vi "InitHardware.vi"(8 "error in (no error)":errorcluster, 11 "ThorLabsCsCamera in":refnum<class "ThorLabsCsCamera.lvclass">) -> (0 "error out":errorcluster, 1 "bit depth":string, 2 "Image Type":T3 items=["Grayscale (U8)", "Grayscale (I16)", "Grayscale (SGL)", "Complex (CSG)", "RGB (U32)", "HSL (U32)", "RGB (U64)", "Grayscale (U16)"], 3 "ThorLabsCsCamera out":refnum<class "ThorLabsCsCamera.lvclass">)   [LabVIEW 2020, in "ThorLabsCsCamera.lvclass"]
uses:
  ThorLabsCsCamera.lvclass
  C:/GEECS/Developers Version/source/Device Drivers/Point Grey Camera/Point Grey Camera.lvclass
  Thorlabs VIs/Controls/Region of Interest.ctl
  Thorlabs VIs/Controls/Binning.ctl
  Point Grey Camera/Point Grey Camera.lvclass/Point Grey Camera.ctl
  ThorLabsCsCamera.lvclass/ThorLabsCsCamera.ctl
  Point Grey Camera/Read Settings 2.vi
  Point Grey Camera/Write Settings 2.vi
  Thorlabs VIs/SubVIs/Parameters Get & Set/Get Parameters/Get ROIAndBin.vi
  Thorlabs VIs/SubVIs/Parameters Get & Set/Get Parameters/Get SensorHeight_pixels.vi
  Thorlabs VIs/SubVIs/Parameters Get & Set/Get Parameters/Get SensorWidth_pixels.vi
  Thorlabs VIs/SubVIs/Parameters Get & Set/Set Parameters/Set ROIAndBin.vi
  Thorlabs VIs/SubVIs/Parameters Get & Set/Get Parameters/Get CameraSensorType.vi
panel:
  out "Binning 2":T1
  out "Region of Interest 2":T2={"Origin - X"=0, "Origin - Y"=0, "Width"=1392, "Height"=1040}
  out "SensorHeight_pixels":u32
  out "SensorWidth_pixels":u32
  out "Binning":T1
  out "Region of Interest":T2={"Origin - X"=0, "Origin - Y"=0, "Width"=1392, "Height"=1040}
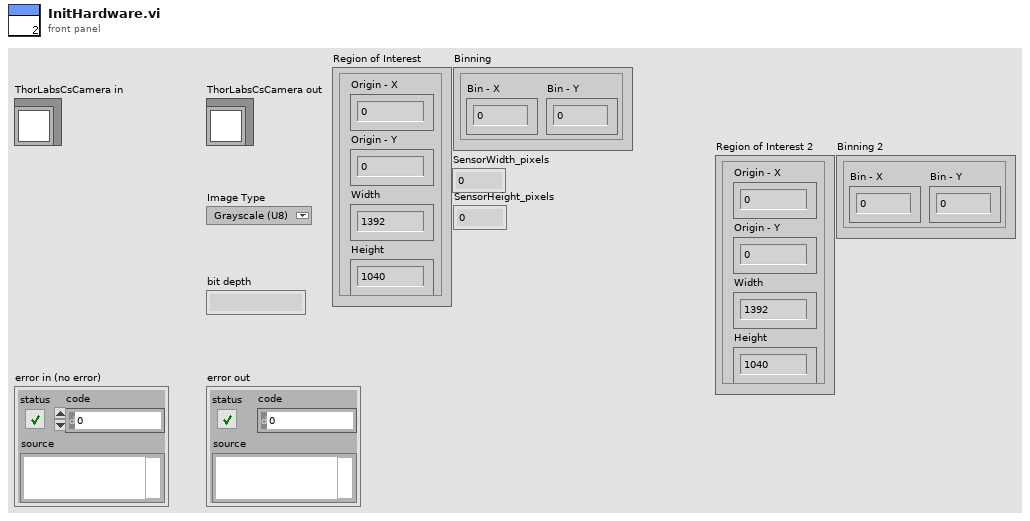
[diagram p1: front panel]
types:
  T1 = typedef "Binning.ctl" = cluster{"Bin - X":u32, "Bin - Y":u32}
  T2 = typedef "Region of Interest.ctl" = cluster{"Origin - X":u32, "Origin - Y":u32, "Width":u32, "Height":u32}
  T3 = typedef "Image Type" = u32
  T4 = typedef "Point Grey Camera.lvclass/SettingsTypdef.ctl" = cluster{"Trigger":T5, "Gain":cluster{"Value":dbl, "Min":dbl, "Max":dbl, "StepSize":dbl, "Tolerance":dbl, "valueactual":dbl}, "Exposure":cluster{"Value":dbl, "Min":dbl, "Max":dbl, "StepSize":dbl, "Tolerance":dbl, "valueactual":dbl}, "Timeout":cluster{"Value":dbl, "Min":dbl, "Max":dbl, "StepSize":dbl, "Tolerance":dbl, "valueactual":dbl}, "LocalSavingPath":path, "Save":T5, "TriggerDelay":cluster{"Value":dbl, "Min":dbl, "Max":dbl, "StepSize":dbl, "Tolerance":dbl, "valueactual":dbl}, "CamSession":string, "ROI":T6, "MaxGUIPixel":cluster{"Value":dbl, "Min":dbl, "Max":dbl, "StepSize":dbl, "Tolerance":dbl, "valueactual":dbl}, "Target":cluster{"X":cluster{"Value":dbl, "Min":dbl, "Max":dbl, "StepSize":dbl, "Tolerance":dbl, "valueactual":dbl}, "Y":cluster{"Value":dbl, "Min":dbl, "Max":dbl, "StepSize":dbl, "Tolerance":dbl, "valueactual":dbl}}, "Analysis":T5, "maxshot#":dbl, "SpatialCalibration":cluster{"Value":dbl, "Min":dbl, "Max":dbl, "StepSize":dbl, "Tolerance":dbl, "valueactual":dbl}, "roistatus":T5, "Lineout":T5, "AnalysisThreshold":cluster{"Value":dbl, "Min":dbl, "Max":dbl, "StepSize":dbl, "Tolerance":dbl, "valueactual":dbl}, "TargetSize":cluster{"X":cluster{"Value":dbl, "Min":dbl, "Max":dbl, "StepSize":dbl, "Tolerance":dbl, "valueactual":dbl}, "Y":cluster{"Value":dbl, "Min":dbl, "Max":dbl, "StepSize":dbl, "Tolerance":dbl, "valueactual":dbl}}, "Simulation":T5, "SpatialCalibrationY":cluster{"Value":dbl, "Min":dbl, "Max":dbl, "StepSize":dbl, "Tolerance":dbl, "valueactual":dbl}, "Target2":cluster{"X":cluster{"Value":dbl, "Min":dbl, "Max":dbl, "StepSize":dbl, "Tolerance":dbl, "valueactual":dbl}, "Y":cluster{"Value":dbl, "Min":dbl, "Max":dbl, "StepSize":dbl, "Tolerance":dbl, "valueactual":dbl}}, "Target2Size":cluster{"X":cluster{"Value":dbl, "Min":dbl, "Max":dbl, "StepSize":dbl, "Tolerance":dbl, "valueactual":dbl}, "Y":cluster{"Value":dbl, "Min":dbl, "Max":dbl, "StepSize":dbl, "Tolerance":dbl, "valueactual":dbl}}, "Crosshair":cluster{"Label1":string, "Label2":string}, "Max2ndMomRadius":cluster{"Value":dbl, "Min":dbl, "Max":dbl, "StepSize":dbl, "Tolerance":dbl, "valueactual":dbl}, "SaveType":T7, "BackgroundPath":path, "GUI8bit":T5, "GUICompression":T5, "CompressionQuality":cluster{"Value":dbl, "Min":dbl, "Max":dbl, "StepSize":dbl, "Tolerance":dbl, "valueactual":dbl}, "SaveAsync":T5, "PerspectivePath":path, "PerspectiveCorrectGUI":T5, "BlackLevel":cluster{"Value":dbl, "Min":dbl, "Max":dbl, "StepSize":dbl, "Tolerance":dbl, "valueactual":dbl}, "TargetBP":cluster{"X":cluster{"Value":dbl, "Min":dbl, "Max":dbl, "StepSize":dbl, "Tolerance":dbl, "valueactual":dbl}, "Y":cluster{"Value":dbl, "Min":dbl, "Max":dbl, "StepSize":dbl, "Tolerance":dbl, "valueactual":dbl}}, "PythonAnalysis":T5, "PythonFunctionName":string, "PythonLineout":T5, "PythonVersion":string, "GEECSBuildsPath":path, "DisplayPythonProcessedImage":T5, "PythonModuleName":string, "AnalysisThresholdHigh":cluster{"Value":dbl, "Min":dbl, "Max":dbl, "StepSize":dbl, "Tolerance":dbl, "valueactual":dbl}, "AnalysisMedianRank":cluster{"Value":dbl, "Min":dbl, "Max":dbl, "StepSize":dbl, "Tolerance":dbl, "valueactual":dbl}, "ClockSpeed":cluster{"Value":dbl, "Min":dbl, "Max":dbl, "StepSize":dbl, "Tolerance":dbl, "valueactual":dbl}, "AutoTrigger":T5, "AutoTriggerLevelMeanCounts":cluster{"Value":dbl, "Min":dbl, "Max":dbl, "StepSize":dbl, "Tolerance":dbl, "valueactual":dbl}, "AnalysisROILeft":cluster{"Value":dbl, "Min":dbl, "Max":dbl, "StepSize":dbl, "Tolerance":dbl, "valueactual":dbl}, "AnalysisROIRight":cluster{"Value":dbl, "Min":dbl, "Max":dbl, "StepSize":dbl, "Tolerance":dbl, "valueactual":dbl}, "AnalysisROITop":cluster{"Value":dbl, "Min":dbl, "Max":dbl, "StepSize":dbl, "Tolerance":dbl, "valueactual":dbl}, "AnalysisROIBottom":cluster{"Value":dbl, "Min":dbl, "Max":dbl, "StepSize":dbl, "Tolerance":dbl, "valueactual":dbl}, "AnalysisROI":T5, "UseSoftwareTrigger":T5, "UDPtrigger":T5, "AutoTriggerLevelMaxCounts":cluster{"Value":dbl, "Min":dbl, "Max":dbl, "StepSize":dbl, "Tolerance":dbl, "valueactual":dbl}}
  T5 = typedef "OnOffTypeDef.ctl" = enum16{"off", "on"}
  T6 = typedef "ROI_TypDef.ctl" = cluster{"Width":cluster{"Value":dbl, "Min":dbl, "Max":dbl, "StepSize":dbl, "Tolerance":dbl, "valueactual":dbl}, "Height":cluster{"Value":dbl, "Min":dbl, "Max":dbl, "StepSize":dbl, "Tolerance":dbl, "valueactual":dbl}, "OffsetX":cluster{"Value":dbl, "Min":dbl, "Max":dbl, "StepSize":dbl, "Tolerance":dbl, "valueactual":dbl}, "OffsetY":cluster{"Value":dbl, "Min":dbl, "Max":dbl, "StepSize":dbl, "Tolerance":dbl, "valueactual":dbl}}
  T7 = typedef "Image save type.ctl" = enum16{"PNG", "BMP", "JPEG", "TDMS", "hdf5"}
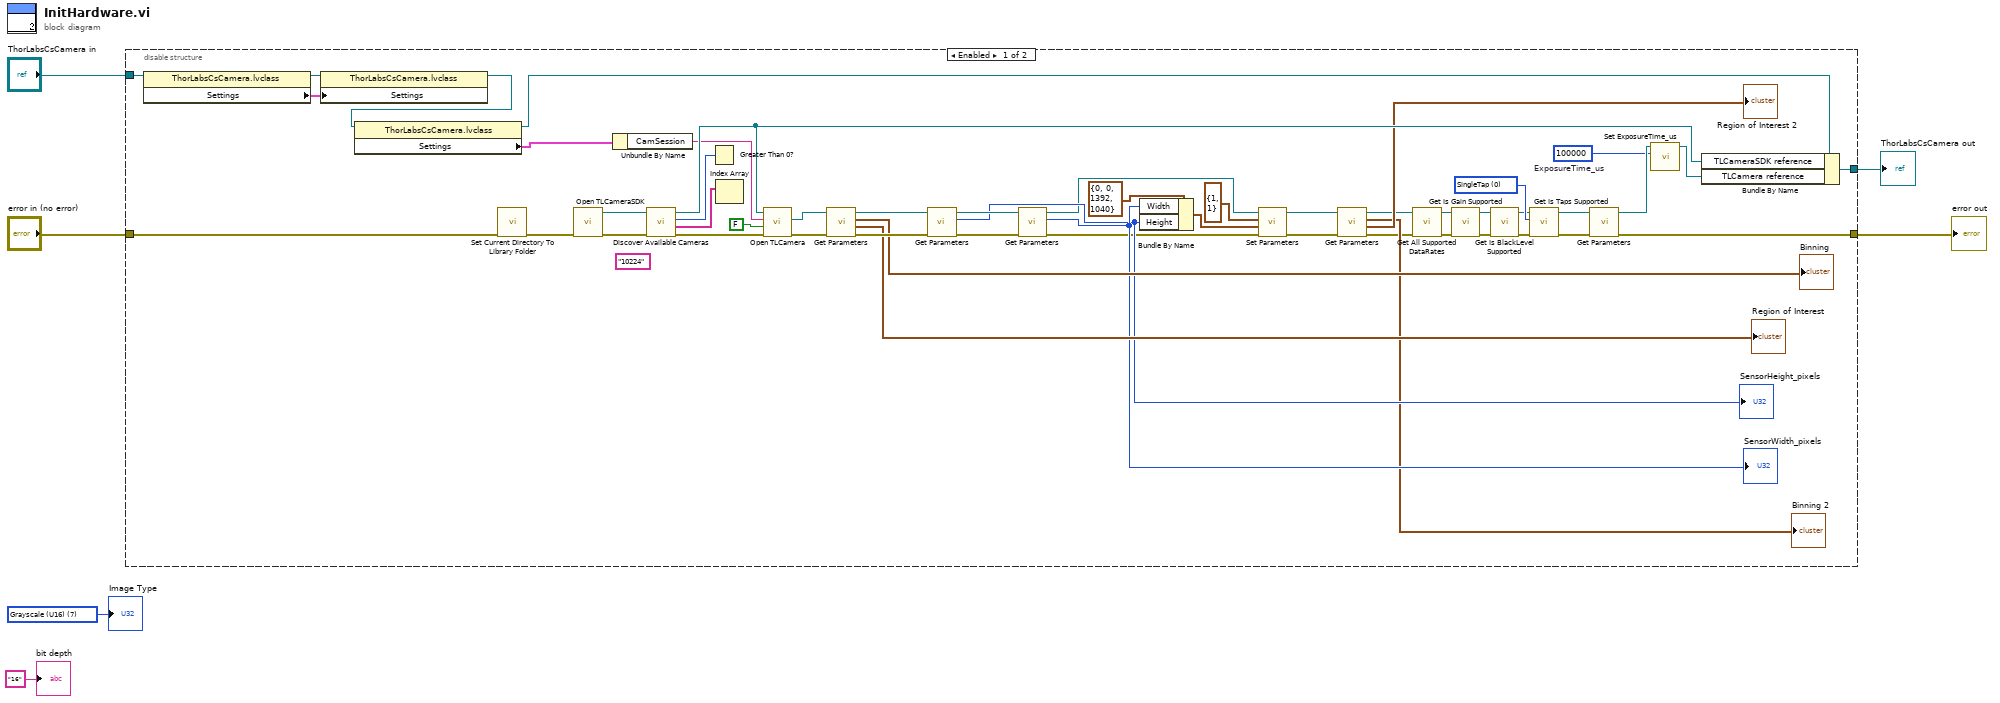
[diagram p0: block diagram]
diagram:
  w1 = T3 7 items=["Grayscale (U8)", "Grayscale (I16)", "Grayscale (SGL)", "Complex (CSG)", "RGB (U32)", "HSL (U32)", "RGB (U64)", "Grayscale (U16)"] ("Image Type")
  n1 = disable-structure shown="Enabled" {
    disable-tunnel: "error in (no error)" -> [w51 w58]
    disable-tunnel: "ThorLabsCsCamera in" -> [w35 w59]
    disable-tunnel: [w30 w59] -> w4
    disable-tunnel: [w29 w58] -> w3
    frame Enabled {
      (unwired) "10224" ("CamSession")
      w26 = u32 100000  # ExposureTime_us
      w44 = 0 items=["SingleTap", "DualTap", "QuadTap"] ("Taps")
      n2 = property class="ThorLabsCsCamera.lvclass"(reference=w35) -> (reference out=w56:refnum<class "ThorLabsCsCamera.lvclass">, "Settings"=w57:T4)  [unwired: 1 in, 1 out]
      n3 = property class="ThorLabsCsCamera.lvclass"(reference=w56, "Settings"=w57) -> (reference out=w9:refnum<class "ThorLabsCsCamera.lvclass">)  [unwired: 1 in, 1 out]
      n4 = property class="ThorLabsCsCamera.lvclass"(reference=w9) -> (reference out=w8:refnum<class "ThorLabsCsCamera.lvclass">, "Settings"=w10:T4)  [unwired: 1 in, 1 out]
      n5 = call "Set Current Directory To Library Folder.vi"("error in (no error)"=w51) -> ("error out"=w52:errorcluster)  [unwired: 10 in]
      n6 = call "Open TLCameraSDK.vi"("error in (no error)"=w52) -> ("error out"=w54:errorcluster, "TLCameraSDK ref out"=w53:refnum<k24>)  [unwired: 9 in]
      n7 = Unbundle By Name(w10) -> ("CamSession"=w7:string)
      n8 = call "Discover Available Cameras.vi"("error in (no error)"=w54, "TLCameraSDK reference"=w53) -> ("error out"=w32:errorcluster, "Serial Numbers"=w36:string[], "Number of Cameras"=w55:i32, "TLCameraSDK reference out"=w34:refnum<k24>)  [unwired: 6 in]
      n9 = Greater Than 0?(x=w55) -> ()  [unwired: 1 out]
      n10 = Index Array(array=w36) -> ()  [unwired: 1 in, 1 out]
      n11 = call "Open TLCamera.vi"("error in (no error)"=w32, "isDiagnosticsMessagesEnabled"=FALSE, "Camera serial number"=w7, "TLCameraSDK reference"=w34) -> ("error out"=w49:errorcluster, "TLCamera reference out"=w48:refnum<k24>)  [unwired: 5 in, 1 out]
      n12 = call-poly "Get Parameters.vi"("error in (no error)"=w49, "TLCamera reference in"=w48) -> ("error out"=w47:errorcluster, "Region of Interest"=→"Region of Interest":T2, "Binning"=→"Binning":T1, "TLCamera reference out"=w45:refnum<k24>)  [unwired: 6 in]
      n13 = call-poly "Get Parameters.vi"("error in (no error)"=w47, "TLCamera reference in"=w45) -> ("error out"=w31:errorcluster, "SensorHeight_pixels"=w21:u32, "TLCamera reference out"=w46:refnum<k24>)  [unwired: 7 in]
      "SensorHeight_pixels" <- w21
      n14 = call-poly "Get Parameters.vi"("error in (no error)"=w31, "TLCamera reference in"=w46) -> ("error out"=w18:errorcluster, "SensorWidth_pixels"=w22:u32, "TLCamera reference out"=w14:refnum<k24>)  [unwired: 7 in]
      "SensorWidth_pixels" <- w22
      n15 = Bundle By Name(cluster=T2 {"Origin - X"=0, "Origin - Y"=0, "Width"=1392, "Height"=1040} ("Region of Interest"), "Width"=w22, "Height"=w21) -> (w19:T2)
      n16 = call-poly "Set Parameters.vi"("error in (no error)"=w18, "Region of Interest"=w19, "Binning"=T1 {"Bin - X"=1, "Bin - Y"=1}, "TLCamera reference in"=w14) -> ("error out"=w12:errorcluster, "TLCamera reference out"=w15:refnum<k24>)  [unwired: 6 in]
      n17 = call-poly "Get Parameters.vi"("error in (no error)"=w12, "TLCamera reference in"=w15) -> ("error out"=w11:errorcluster, "Region of Interest"=→"Region of Interest 2":T2, "Binning"=→"Binning 2":T1, "TLCamera reference out"=w13:refnum<k24>)  [unwired: 6 in]
      n18 = call "Get All Supported DataRates.vi"("error in (no error)"=w11, "TLCamera reference"=w13) -> ("error out"=w43:errorcluster, "TLCamera reference out"=w40:refnum<k24>)  [unwired: 7 in, 1 out]
      n19 = call "Get Is Gain Supported.vi"("error in (no error)"=w43, "TLCamera reference in"=w40) -> ("error out"=w39:errorcluster, "TLCamera reference out"=w38:refnum<k24>)  [unwired: 7 in, 1 out]
      n20 = call "Get Is BlackLevel Supported.vi"("error in (no error)"=w39, "TLCamera reference in"=w38) -> ("error out"=w33:errorcluster, "TLCamera reference out"=w37:refnum<k24>)  [unwired: 7 in, 1 out]
      n21 = call "Get Is Taps Supported.vi"("error in (no error)"=w33, "Taps"=w44, "TLCamera reference"=w37) -> ("error out"=w42:errorcluster, "TLCamera reference out"=w41:refnum<k24>)  [unwired: 6 in, 1 out]
      n22 = call-poly "Get Parameters.vi"("error in (no error)"=w42, "TLCamera reference in"=w41) -> ("error out"=w29:errorcluster, "TLCamera reference out"=w28:refnum<k24>)  [unwired: 7 in, 1 out]
      n23 = call "Set ExposureTime_us.vi"("ExposureTime_us"=w26, "TLCamera reference in"=w28) -> ("TLCamera reference out"=w27:refnum<k24>)  [unwired: 8 in, 1 out]
      n24 = Bundle By Name(cluster=w8, "TLCameraSDK reference"=w34, "TLCamera reference"=w27) -> (w30:refnum<class "ThorLabsCsCamera.lvclass">)
    }
    frame Disabled {
    }
  }
  "ThorLabsCsCamera out" <- w4
  "error out" <- w3
  "Image Type" <- w1
  "bit depth" <- "16" ("bit depth")
